vi "IsValidDataBitrate.vi"(11 "Bit Rate":i32) -> (3 "x >= 0?":bool)   [LabVIEW 2026]
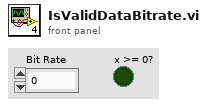
[diagram p1: front panel]
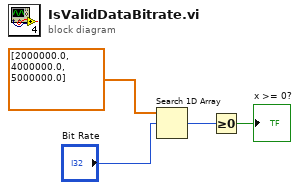
[diagram p0: block diagram]
diagram:
  n1 = Search 1D Array(1D array=dbl[] [2000000.0, 4000000.0, 5000000.0], element="Bit Rate") -> (index of element=w2:i32)  [unwired: 1 in]
  n2 = Greater Or Equal To 0?(x=w2) -> (x >= 0?=→"x >= 0?":bool)
